vi "gamepad_control.vi"(0 "device ID in":refnum<k1>, 1 "preskaler 2":dbl=10.0, 5 "scansize [nm]":refnum<vi>, 7 "scanstart [nm]":refnum<vi>, 9 "read":i64[](array[numeric]), 11 "error in (no error)":errorcluster, 12 "dynamika [nm/s]":refnum<vi>) -> (3 "preskaler":dbl=10.0, 4 "Refnum out":refnum<k1>, 6 "START":bool, 8 "appended array":bool[](array[boolean]), 10 "SAVE":bool, 15 "error out":errorcluster)   [LabVIEW 2013]
uses:
  <vilib>/Utility/inputDevices.llb/joystickAcquire.vi
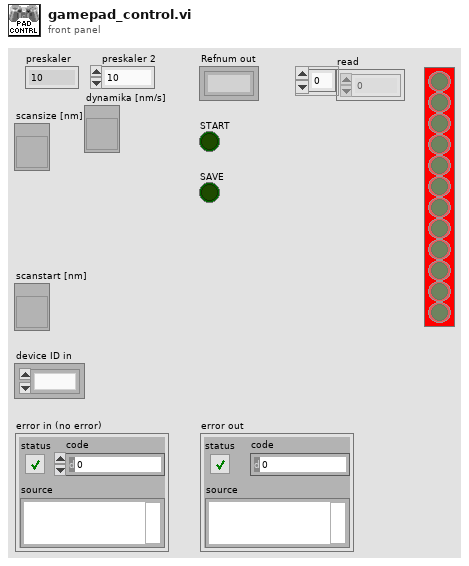
[diagram p1: front panel]
types:
  T1 = cluster{"button 1":bool, "button 2":bool, "button 3":bool, "button 4":bool, "button 5":bool, "button 6":bool, "button 7":bool, "button 8":bool, "button 9":bool, "button 10":bool, "button 11":bool, "button 12":bool, "button 13":bool, "button 14":bool, "button 15":bool, "button 16":bool, "button 17":bool, "button 18":bool, "button 19":bool, "button 20":bool, "button 21":bool, "button 22":bool, "button 23":bool, "button 24":bool, "button 25":bool, "button 26":bool, "button 27":bool, "button 28":bool, "button 29":bool, "button 30":bool, "button 31":bool, "button 32":bool}
  T2 = cluster{"pov 1":i32, "pov 2":i32, "pov 3":i32, "pov 4":i32}
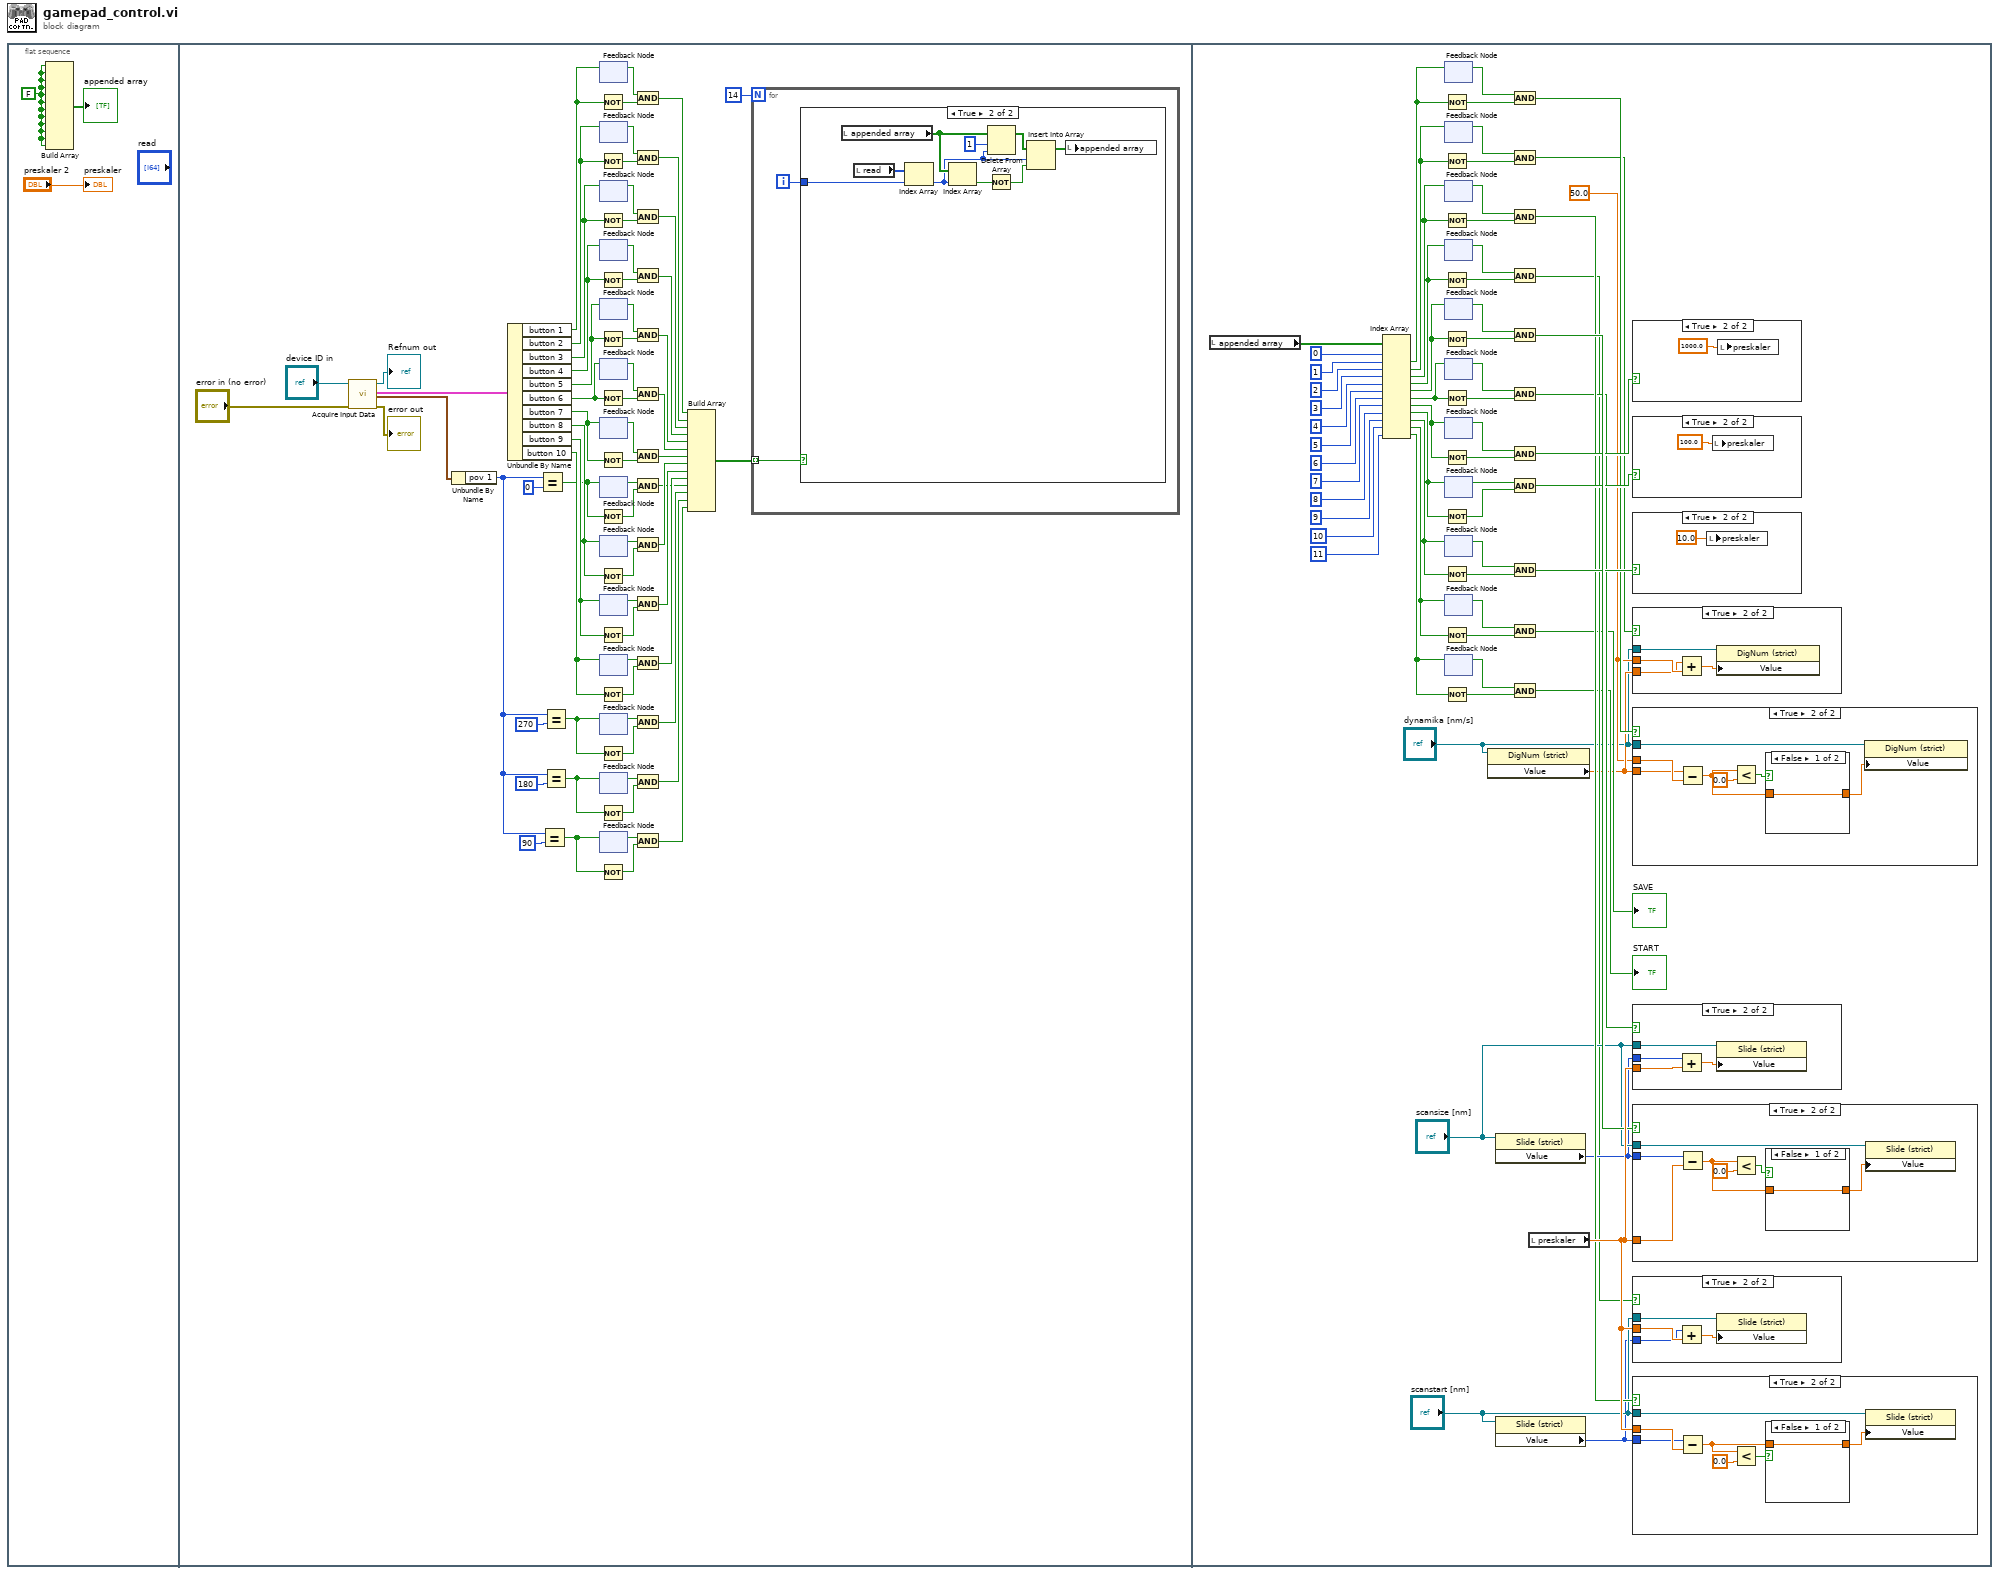
[diagram p0: block diagram]
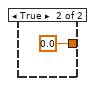
[diagram p4: hidden frame]
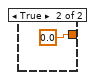
[diagram p10: hidden frame]
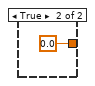
[diagram p13: hidden frame]
diagram:
  n1 = flat-sequence {
    frame #0 {
      w1 = FALSE ("x .xor. y?")
      n2 = Build Array(w1, w1, w1, w1, w1, w1, w1, w1, w1, w1, w1, w1) -> (→"appended array":bool[])
      "preskaler" <- "preskaler 2"
    }
    frame #1 {
      n3 = call-poly <vilib>:"Acquire Input Data.vi"("device ID"="device ID in", "error in (no error)"="error in (no error)") -> ("device ID"=→"Refnum out":refnum<k1>, "button info"=w71:T1, "direction info"=w72:T2, "error out"=→"error out":errorcluster)  [unwired: 13 in, 1 out]
      n4 = Unbundle By Name(w72) -> ("pov 1"=w68:i32)
      n5 = Unbundle By Name(w71) -> ("button 1"=w31:bool, "button 2"=w30:bool, "button 3"=w29:bool, "button 4"=w28:bool, "button 5"=w27:bool, "button 6"=w26:bool, "button 7"=w25:bool, "button 8"=w24:bool, "button 9"=w23:bool, "button 10"=w22:bool)
      n6 = Equal?(x=w68, y=0) -> (x = y?=w21:bool)
      n7 = Equal?(x=w68, y=90) -> (x = y?=w18:bool)
      n8 = Equal?(x=w68, y=270) -> (x = y?=w20:bool)
      n9 = Equal?(x=w68, y=180) -> (x = y?=w19:bool)
      n10 = Not(x=w31) -> (.not. x?=w57:bool)
      n11 = Not(x=w30) -> (.not. x?=w54:bool)
      n12 = Not(x=w29) -> (.not. x?=w53:bool)
      n13 = Not(x=w28) -> (.not. x?=w50:bool)
      n14 = Not(x=w27) -> (.not. x?=w49:bool)
      n15 = Not(x=w26) -> (.not. x?=w46:bool)
      n16 = Not(x=w25) -> (.not. x?=w45:bool)
      n17 = Not(x=w21) -> (.not. x?=w38:bool)
      n18 = Not(x=w24) -> (.not. x?=w42:bool)
      n19 = Not(x=w23) -> (.not. x?=w41:bool)
      n20 = Not(x=w22) -> (.not. x?=w58:bool)
      n21 = Not(x=w20) -> (.not. x?=w37:bool)
      n22 = Not(x=w19) -> (.not. x?=w34:bool)
      n23 = Not(x=w18) -> (.not. x?=w33:bool)
      n24 = feedback #1() -> (w56:bool)  [unwired: 1 in]
      n25 = feedback-in #1(w31) -> ()
      n26 = feedback #2() -> (w55:bool)  [unwired: 1 in]
      n27 = feedback-in #2(w30) -> ()
      n28 = feedback #3() -> (w52:bool)  [unwired: 1 in]
      n29 = feedback-in #3(w29) -> ()
      n30 = feedback #4() -> (w51:bool)  [unwired: 1 in]
      n31 = feedback-in #4(w28) -> ()
      n32 = feedback #5() -> (w48:bool)  [unwired: 1 in]
      n33 = feedback-in #5(w27) -> ()
      n34 = feedback #6() -> (w47:bool)  [unwired: 1 in]
      n35 = feedback-in #6(w26) -> ()
      n36 = feedback #7() -> (w44:bool)  [unwired: 1 in]
      n37 = feedback-in #7(w25) -> ()
      n38 = feedback #8() -> (w39:bool)  [unwired: 1 in]
      n39 = feedback-in #8(w21) -> ()
      n40 = feedback #9() -> (w43:bool)  [unwired: 1 in]
      n41 = feedback-in #9(w24) -> ()
      n42 = feedback #10() -> (w40:bool)  [unwired: 1 in]
      n43 = feedback-in #10(w23) -> ()
      n44 = feedback #11() -> (w59:bool)  [unwired: 1 in]
      n45 = feedback-in #11(w22) -> ()
      n46 = feedback #12() -> (w36:bool)  [unwired: 1 in]
      n47 = feedback-in #12(w20) -> ()
      n48 = feedback #13() -> (w35:bool)  [unwired: 1 in]
      n49 = feedback-in #13(w19) -> ()
      n50 = feedback #14() -> (w32:bool)  [unwired: 1 in]
      n51 = feedback-in #14(w18) -> ()
      n52 = And(x=w56, y=w57) -> (x .and. y?=w17:bool)
      n53 = And(x=w55, y=w54) -> (x .and. y?=w16:bool)
      n54 = And(x=w52, y=w53) -> (x .and. y?=w15:bool)
      n55 = And(x=w51, y=w50) -> (x .and. y?=w14:bool)
      n56 = And(x=w48, y=w49) -> (x .and. y?=w13:bool)
      n57 = And(x=w47, y=w46) -> (x .and. y?=w12:bool)
      n58 = And(x=w44, y=w45) -> (x .and. y?=w11:bool)
      n59 = And(x=w39, y=w38) -> (x .and. y?=w7:bool)
      n60 = And(x=w43, y=w42) -> (x .and. y?=w10:bool)
      n61 = And(x=w40, y=w41) -> (x .and. y?=w9:bool)
      n62 = And(x=w59, y=w58) -> (x .and. y?=w8:bool)
      n63 = And(x=w36, y=w37) -> (x .and. y?=w6:bool)
      n64 = And(x=w35, y=w34) -> (x .and. y?=w5:bool)
      n65 = And(x=w32, y=w33) -> (x .and. y?=w4:bool)
      n66 = Build Array(w17, w16, w15, w14, w13, w12, w11, w10, w9, w8, w7, w6, w5, w4) -> (w69:bool[])
      n67 = for {
        N: 14 -> [_]
        tunnel: w69 -> [w74] mode=indexing
        i -> [w73]
        n68 = case shown="True" w74 {
          tunnel: w73 -> [_ w80]
          frame False {
          }
          frame True {
            n69 = local read "appended array"() -> (w78:bool[])
            n70 = local read "read"() -> (w79:i64[])
            n71 = Index Array(array=w79, index=w80) -> (element=w77:i64)
            n72 = Index Array(array=w78, index=w77) -> (element=w76:bool)
            n73 = Not(x=w76) -> (.not. x?=w75:bool)
            n74 = Delete From Array(array=w78, length=1, index=w77) -> (array with subset deleted=w82:bool[])  [unwired: 1 out]
            n75 = Insert Into Array(array=w82, index=w77, new element=w75) -> (w81:bool[])
            n76 = local write "appended array"(w81) -> ()
          }
        }
      }
    }
    frame #2 {
      w122 = 50.0 ("preskaler 4")
      n77 = local read "appended array"() -> (w119:bool[])
      n78 = Index Array(array=w119, index #1=0 ("index"), index #2=1 ("index"), index #3=2 ("index"), index #4=3 ("index"), index #5=4 ("index"), index #6=5 ("index"), index #7=6 ("index"), index #8=7 ("index"), index #9=8 ("index"), index #10=9 ("index"), index #11=10 ("index"), index #12=11 ("index")) -> (element #2=w85:bool, element #3=w84:bool, element #4=w103:bool, element #5=w101:bool, element #6=w99:bool, element #7=w97:bool, element #8=w95:bool, element #9=w92:bool, element #10=w90:bool, element #11=w89:bool, element #12=w87:bool)  [unwired: 1 out]
      n79 = Not(x=w85) -> (.not. x?=w120:bool)
      n80 = Not(x=w84) -> (.not. x?=w105:bool)
      n81 = Not(x=w103) -> (.not. x?=w137:bool)
      n82 = Not(x=w101) -> (.not. x?=w138:bool)
      n83 = Not(x=w99) -> (.not. x?=w146:bool)
      n84 = Not(x=w97) -> (.not. x?=w147:bool)
      n85 = Not(x=w95) -> (.not. x?=w142:bool)
      n86 = Not(x=w92) -> (.not. x?=w143:bool)
      n87 = Not(x=w90) -> (.not. x?=w144:bool)
      n88 = Not(x=w89) -> (.not. x?=w128:bool)
      n89 = Not(x=w87) -> (.not. x?=w129:bool)
      n90 = feedback #15() -> (w104:bool)  [unwired: 1 in]
      n91 = feedback-in #15(w85) -> ()
      n92 = feedback #16() -> (w106:bool)  [unwired: 1 in]
      n93 = feedback-in #16(w84) -> ()
      n94 = feedback #17() -> (w102:bool)  [unwired: 1 in]
      n95 = feedback-in #17(w103) -> ()
      n96 = feedback #18() -> (w100:bool)  [unwired: 1 in]
      n97 = feedback-in #18(w101) -> ()
      n98 = feedback #19() -> (w98:bool)  [unwired: 1 in]
      n99 = feedback-in #19(w99) -> ()
      n100 = feedback #20() -> (w96:bool)  [unwired: 1 in]
      n101 = feedback-in #20(w97) -> ()
      n102 = feedback #21() -> (w94:bool)  [unwired: 1 in]
      n103 = feedback-in #21(w95) -> ()
      n104 = feedback #22() -> (w93:bool)  [unwired: 1 in]
      n105 = feedback-in #22(w92) -> ()
      n106 = feedback #23() -> (w91:bool)  [unwired: 1 in]
      n107 = feedback-in #23(w90) -> ()
      n108 = feedback #24() -> (w88:bool)  [unwired: 1 in]
      n109 = feedback-in #24(w89) -> ()
      n110 = feedback #25() -> (w86:bool)  [unwired: 1 in]
      n111 = feedback-in #25(w87) -> ()
      n112 = property class="DigNum (strict)"(reference="dynamika [nm/s]") -> ("Value"=w124:dbl)  [unwired: 1 in, 2 out]
      n113 = property class="Slide (strict)"(reference="scansize [nm]") -> ("Value"=w132:i64)  [unwired: 1 in, 2 out]
      n114 = property class="Slide (strict)"(reference="scanstart [nm]") -> ("Value"=w134:i64)  [unwired: 1 in, 2 out]
      n115 = And(x=w104, y=w120) -> (x .and. y?=w125:bool)
      n116 = And(x=w106, y=w105) -> (x .and. y?=w123:bool)
      n117 = And(x=w102, y=w137) -> (x .and. y?=w136:bool)
      n118 = And(x=w100, y=w138) -> (x .and. y?=w130:bool)
      n119 = And(x=w98, y=w146) -> (x .and. y?=w145:bool)
      n120 = And(x=w96, y=w147) -> (x .and. y?=w131:bool)
      n121 = And(x=w94, y=w142) -> (x .and. y?=w139:bool)
      n122 = And(x=w93, y=w143) -> (x .and. y?=w140:bool)
      n123 = And(x=w91, y=w144) -> (x .and. y?=w141:bool)
      n124 = And(x=w88, y=w128) -> (x .and. y?=→"SAVE":bool)
      n125 = And(x=w86, y=w129) -> (x .and. y?=→"START":bool)
      n126 = local read "preskaler"() -> (w148:dbl)
      n127 = case shown="True" w139 {
        frame False {
        }
        frame True {
          n128 = local write "preskaler"(1000.0 ("preskaler")) -> ()
        }
      }
      n129 = case shown="True" w140 {
        frame False {
        }
        frame True {
          n130 = local write "preskaler"(100.0 ("preskaler")) -> ()
        }
      }
      n131 = case shown="True" w141 {
        frame False {
        }
        frame True {
          n132 = local write "preskaler"(10.0 ("preskaler")) -> ()
        }
      }
      n133 = case shown="True" w123 {
        tunnel: w122 -> [_ w160]
        tunnel: "dynamika [nm/s]" -> [_ w159]
        tunnel: w124 -> [_ w158]
        frame False {
        }
        frame True {
          n134 = Add(x=w158, y=w160) -> (x+y=w161:dbl)
          n135 = property class="DigNum (strict)"(reference=w159, "Value"=w161) -> ()  [unwired: 1 in, 2 out]
        }
      }
      n136 = case shown="True" w125 {
        tunnel: w122 -> [_ w155]
        tunnel: "dynamika [nm/s]" -> [_ w154]
        tunnel: w124 -> [_ w153]
        frame False {
        }
        frame True {
          n137 = Subtract(x=w153, y=w155) -> (x-y=w150:dbl)
          n138 = Less?(x=w150, y=0.0) -> (x < y?=w152:bool)
          n139 = case shown="False" w152 {
            tunnel: [w156 0.0 ("y")] -> w149
            tunnel: w150 -> [w156 _]
            frame False {
            }
            frame True {
            }
          }
          n140 = property class="DigNum (strict)"(reference=w154, "Value"=w149) -> ()  [unwired: 1 in, 2 out]
        }
      }
      n141 = case shown="True" w131 {
        tunnel: w148 -> [_ w176]
        tunnel: "scansize [nm]" -> [_ w175]
        tunnel: w132 -> [_ w174]
        frame False {
        }
        frame True {
          n142 = Add(x=w174, y=w176) -> (x+y=w177:dbl)
          n143 = property class="Slide (strict)"(reference=w175, "Value"=w177) -> ()  [unwired: 1 in, 2 out]
        }
      }
      n144 = case shown="True" w145 {
        tunnel: w148 -> [_ w184]
        tunnel: "scansize [nm]" -> [_ w183]
        tunnel: w132 -> [_ w182]
        frame False {
        }
        frame True {
          n145 = Subtract(x=w182, y=w184) -> (x-y=w179:dbl)
          n146 = Less?(x=w179, y=0.0) -> (x < y?=w181:bool)
          n147 = case shown="False" w181 {
            tunnel: [w185 0.0 ("y")] -> w178
            tunnel: w179 -> [w185 _]
            frame False {
            }
            frame True {
            }
          }
          n148 = property class="Slide (strict)"(reference=w183, "Value"=w178) -> ()  [unwired: 1 in, 2 out]
        }
      }
      n149 = case shown="True" w130 {
        tunnel: w148 -> [_ w189]
        tunnel: "scanstart [nm]" -> [_ w188]
        tunnel: w134 -> [_ w187]
        frame False {
        }
        frame True {
          n150 = Add(x=w187, y=w189) -> (x+y=w190:dbl)
          n151 = property class="Slide (strict)"(reference=w188, "Value"=w190) -> ()  [unwired: 1 in, 2 out]
        }
      }
      n152 = case shown="True" w136 {
        tunnel: w148 -> [_ w171]
        tunnel: "scanstart [nm]" -> [_ w170]
        tunnel: w134 -> [_ w169]
        frame False {
        }
        frame True {
          n153 = Subtract(x=w169, y=w171) -> (x-y=w166:dbl)
          n154 = Less?(x=w166, y=0.0) -> (x < y?=w168:bool)
          n155 = case shown="False" w168 {
            tunnel: [w172 0.0 ("y")] -> w165
            tunnel: w166 -> [w172 _]
            frame False {
            }
            frame True {
            }
          }
          n156 = property class="Slide (strict)"(reference=w170, "Value"=w165) -> ()  [unwired: 1 in, 2 out]
        }
      }
    }
  }
